vi "VelocityPlots.vi"(7 "Reset":bool, 8 "Nu_d":dbl[](array[numeric])=[0.0, 0.0, 0.0, 0.0, 0.0, 0.0], 9 "Nu_e":dbl[](array[numeric])=[0.0, 0.0, 0.0, 0.0, 0.0, 0.0], 10 "Nu":dbl[](array[numeric])=[0.0, 0.0, 0.0, 0.0, 0.0, 0.0]) -> ()   [LabVIEW 2014]
panel:
  out "p":T1(graph)
  out "q":T1(graph)
  out "v":T1(graph)
  out "u":T1(graph)
  out "r":T1(graph)
  out "w":T1(graph)
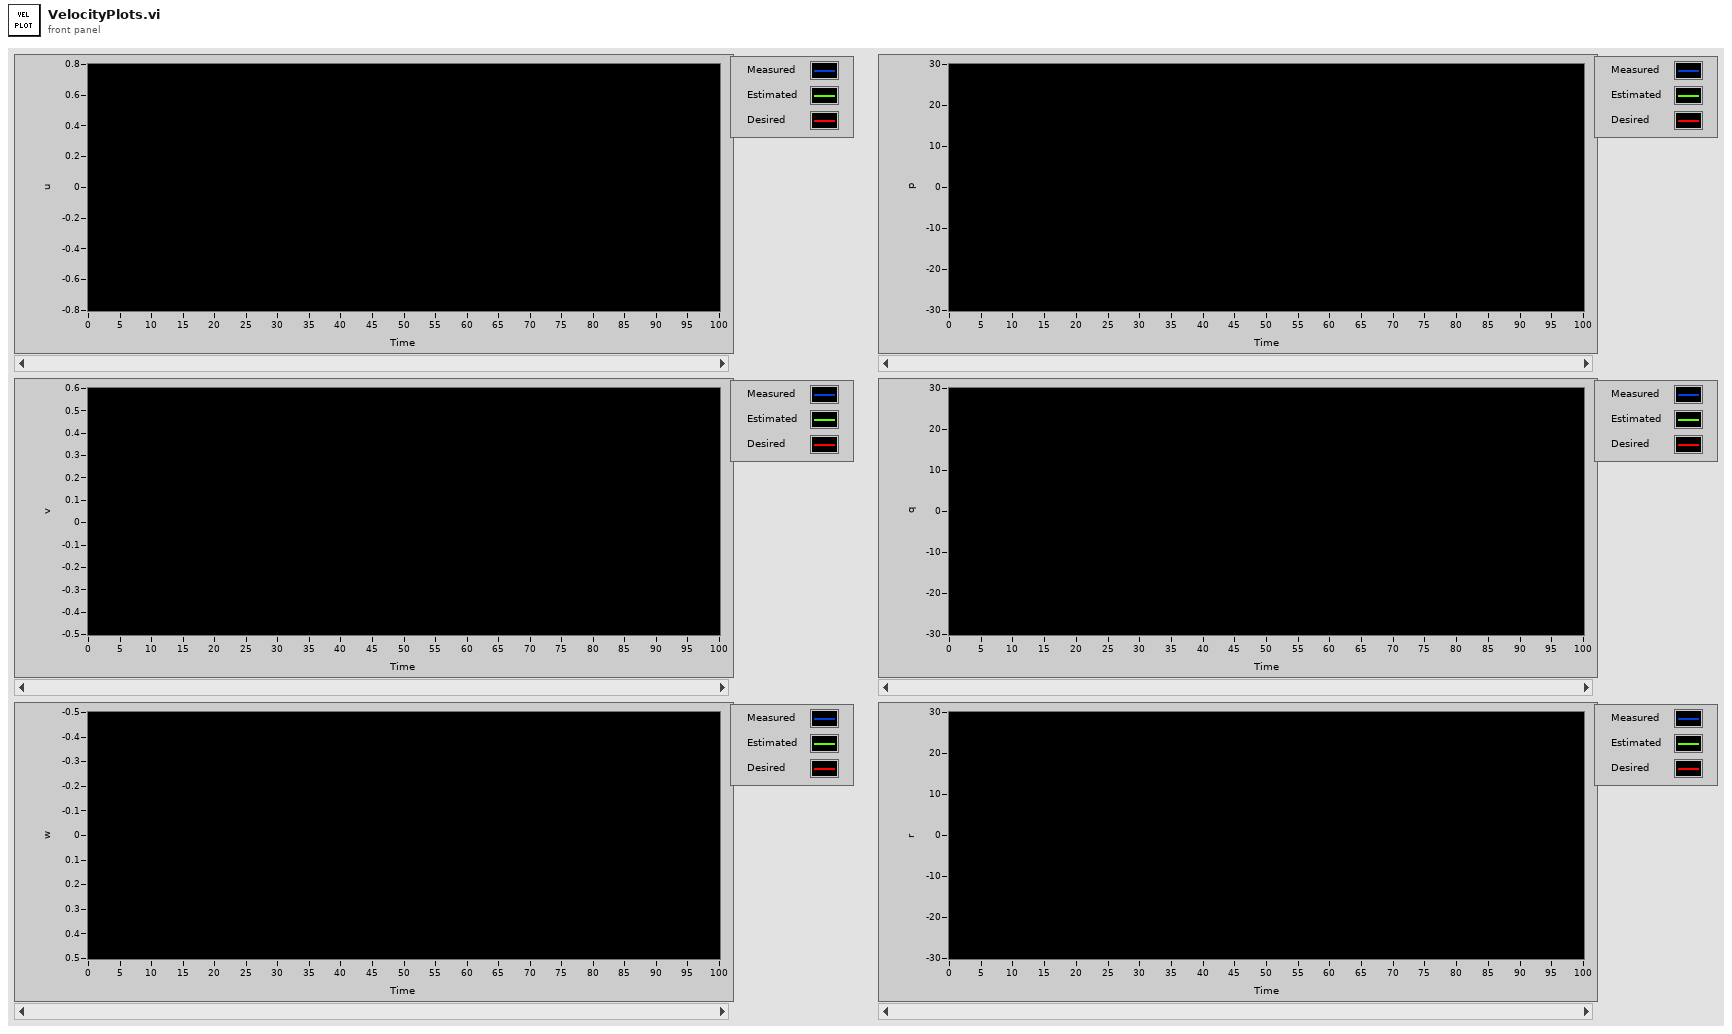
[diagram p1: front panel]
types:
  T1 = cluster{"Numeric":dbl, "Numeric":dbl, "Numeric":dbl}
  T2 = cluster{"Numeric":dbl, "Numeric":dbl, "Numeric":dbl}[]
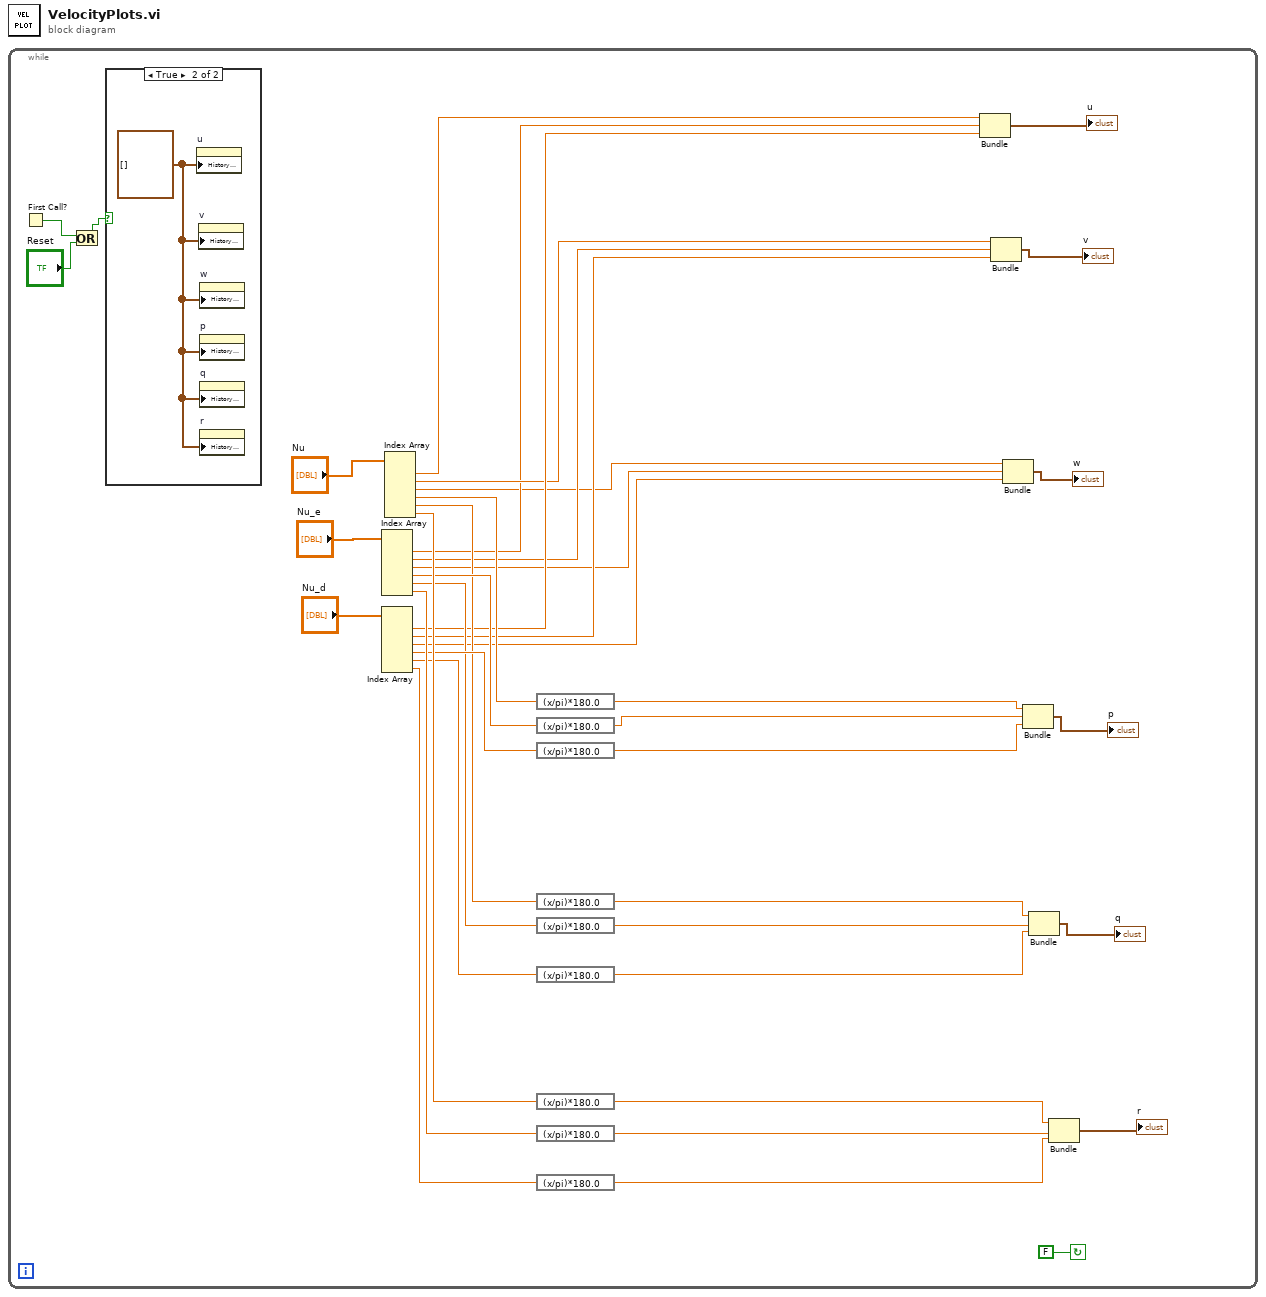
[diagram p0: block diagram]
diagram:
  n1 = while {
    stop <- FALSE continue-if-true
    n2 = First Call?() -> (First Call?: T/F=w2:bool)
    n3 = Or(x=w2, y="Reset") -> (x .or. y?=w1:bool)
    n4 = case shown="True" w1 {
      frame False {
      }
      frame True {
        w41 = T2 [] ("History Data")
        n5 = property on="u" class="WFChart (strict)"("History Data"=w41) -> ()  [unwired: 2 in, 2 out]
        n6 = property on="v" class="WFChart (strict)"("History Data"=w41) -> ()  [unwired: 2 in, 2 out]
        n7 = property on="w" class="WFChart (strict)"("History Data"=w41) -> ()  [unwired: 2 in, 2 out]
        n8 = property on="p" class="WFChart (strict)"("History Data"=w41) -> ()  [unwired: 2 in, 2 out]
        n9 = property on="q" class="WFChart (strict)"("History Data"=w41) -> ()  [unwired: 2 in, 2 out]
        n10 = property on="r" class="WFChart (strict)"("History Data"=w41) -> ()  [unwired: 2 in, 2 out]
      }
    }
    n11 = Index Array(array="Nu_e") -> (element #1=w24:dbl, element #2=w23:dbl, element #3=w20:dbl, element #4=w36:dbl, element #5=w33:dbl, element #6=w39:dbl)  [unwired: 6 in]
    n12 = Index Array(array="Nu_d") -> (element #1=w26:dbl, element #2=w22:dbl, element #3=w19:dbl, element #4=w35:dbl, element #5=w32:dbl, element #6=w38:dbl)  [unwired: 6 in]
    n13 = Index Array(array="Nu") -> (element #1=w27:dbl, element #2=w25:dbl, element #3=w21:dbl, element #4=w37:dbl, element #5=w34:dbl, element #6=w40:dbl)  [unwired: 6 in]
    n14 = expression code="(x/pi)*180.0" ("radians to degrees")(w37) -> (w18:dbl)
    n15 = expression code="(x/pi)*180.0" ("radians to degrees")(w36) -> (w17:dbl)
    n16 = expression code="(x/pi)*180.0" ("radians to degrees")(w35) -> (w16:dbl)
    n17 = expression code="(x/pi)*180.0" ("radians to degrees")(w34) -> (w15:dbl)
    n18 = expression code="(x/pi)*180.0" ("radians to degrees")(w33) -> (w14:dbl)
    n19 = expression code="(x/pi)*180.0" ("radians to degrees")(w32) -> (w13:dbl)
    n20 = expression code="(x/pi)*180.0" ("radians to degrees")(w40) -> (w12:dbl)
    n21 = expression code="(x/pi)*180.0" ("radians to degrees")(w39) -> (w11:dbl)
    n22 = expression code="(x/pi)*180.0" ("radians to degrees")(w38) -> (w10:dbl)
    n23 = Bundle("Numeric"=w27, "Numeric"=w24, "Numeric"=w26) -> (→"u":T1)  [unwired: 1 in]
    n24 = Bundle("Numeric"=w25, "Numeric"=w23, "Numeric"=w22) -> (→"v":T1)  [unwired: 1 in]
    n25 = Bundle("Numeric"=w21, "Numeric"=w20, "Numeric"=w19) -> (→"w":T1)  [unwired: 1 in]
    n26 = Bundle("Numeric"=w18, "Numeric"=w17, "Numeric"=w16) -> (→"p":T1)  [unwired: 1 in]
    n27 = Bundle("Numeric"=w15, "Numeric"=w14, "Numeric"=w13) -> (→"q":T1)  [unwired: 1 in]
    n28 = Bundle("Numeric"=w12, "Numeric"=w11, "Numeric"=w10) -> (→"r":T1)  [unwired: 1 in]
  }
